vi "camera-write_trigger-mode-frame-start.vi"(6 "error in (no error)":errorcluster, 8 "Option":enum16{"Off", "On"}(ring), 9 "IMAQ Session In":refnum<k11>) -> (0 "error out":errorcluster, 1 "Data":string, 2 "Address":string, 3 "IMAQ Session Out":refnum<k11>)   [LabVIEW 2012]
panel:
  out "Loop Iteration":i32
  out "ACK/NAK":string
  out "String to Write":string
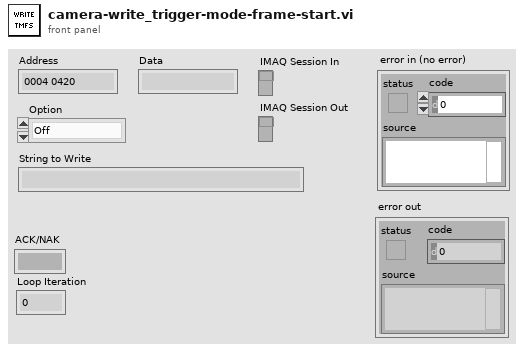
[diagram p1: front panel]
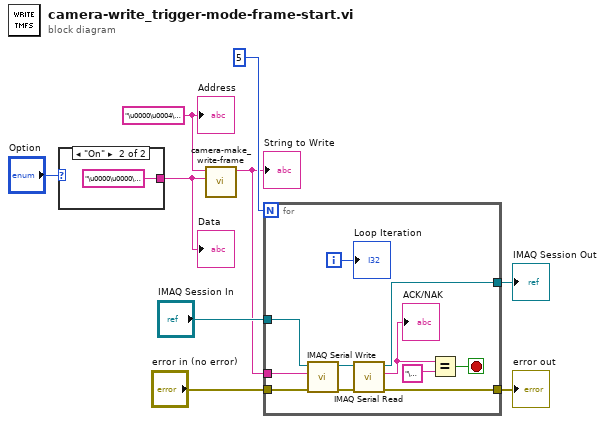
[diagram p0: block diagram]
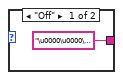
[diagram p2: hidden frame]
diagram:
  w9 = "\u0000\u0004\u0002\u0000" ("Address")
  n1 = case shown="\"On\"" "Option" {
    tunnel: ["\u0000\u0000\u0000\u0000" ("Address") "\u0000\u0000\u0000\u0001" ("Address")] -> w1
    frame "Off" {
    }
    frame "On" {
    }
  }
  "Data" <- w1
  n2 = call "camera-make_write-frame.vi"("Data"=w1, "Address"=w9) -> ("Serial String"=w6:string)  [unwired: 9 in]
  "String to Write" <- w6
  n3 = for {
    N: 5 -> [_]
    tunnel: "IMAQ Session In" -> [w22]
    tunnel: w6 -> [w21]
    tunnel: [w20] -> w5
    tunnel: "error in (no error)" -> [w19]
    tunnel: [w17] -> w3
    i -> [w13]
    stop <- w16 stop-if-true
    n4 = call <vilib>:"IMAQ Serial Write.vi"("error in (no error)"=w19, "String to write"=w21, "IMAQ Session In"=w22) -> ("error out"=w18:errorcluster, "IMAQ Session Out"=w12:refnum<k11>)  [unwired: 5 in]
    n5 = call <vilib>:"IMAQ Serial Read.vi"("error in (no error)"=w18, "IMAQ Session In"=w12) -> ("error out"=w17:errorcluster, "String Read"=w15:string, "IMAQ Session Out"=w20:refnum<k11>)  [unwired: 4 in, 1 out]
    "ACK/NAK" <- w15
    n6 = Equal?(x=w15, y="\u0006") -> (x = y?=w16:bool)
    "Loop Iteration" <- w13
  }
  "IMAQ Session Out" <- w5
  "error out" <- w3
  "Address" <- w9
